vi "Read SSH.vi"(8 "Error In":errorcluster, 11 "Known Hosts In":refnum<class "Known Hosts.lvclass">) -> (0 "Error Out":errorcluster, 2 "SSH":refnum<class "SSH.lvclass">, 3 "Known Hosts Out":refnum<class "Known Hosts.lvclass">)   [LabVIEW 2021, in "Field_RnD_Services_LIBSSH2_Toolkit.lvlib" / "Known Hosts.lvclass"]
doc: "Gets the SSH context used to create this Known Hosts object and corresponding internal libssh2lv shared library linked list."
uses:
  Known Hosts.lvclass
  SSH/SSH.lvclass
  Known Hosts.lvclass/Known Hosts.ctl
  Session/Session.lvclass
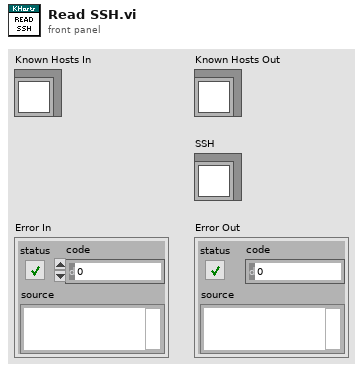
[diagram p1: front panel]
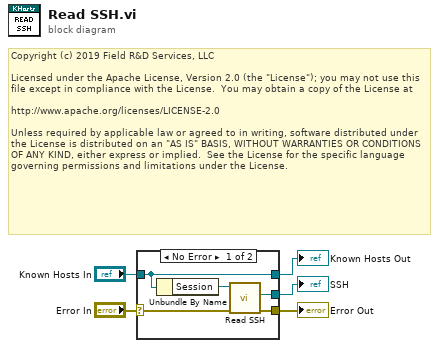
[diagram p0: block diagram]
diagram:
  # "Copyright (c) 2019 Field R&D Services, LLC\n\nLicensed under the Apache License, Version 2.0 (the \"License\"); you may not use this file except in compliance with the License.  You may obtain a copy of the License at\n\nhttp://www.apache.org/licenses/LICENSE-2.0\n\nUnless required by applicable law or agreed to in writing, software distributed under the License is distributed on an \"AS IS\" BASIS, WITHOUT WARRANTIES OR CONDITIONS OF ANY KIND, either express or implied.  See the License for the specific language governing permissions and limitations under the License."
  n1 = case shown="No Error" "Error In" {
    selector: "Error In" -> [w8 w11]
    tunnel: "Known Hosts In" -> [w10 w12]
    tunnel: [w10 w12] -> w3
    tunnel: [w6 w11] -> w2
    tunnel: [w7 _] -> w1
    frame No Error {
      n2 = Unbundle By Name(w10) -> ("Session"=w9:refnum<class "Session.lvclass">)
      n3 = call "Read SSH.vi"("Error In"=w8, "Session In"=w9) -> ("Erorr Out"=w6:errorcluster, "SSH"=w7:refnum<class "SSH.lvclass">)  [unwired: 7 in, 1 out]
    }
    frame Error {
    }
  }
  "Known Hosts Out" <- w3
  "Error Out" <- w2
  "SSH" <- w1
